vi "GEA3 Get ERD Info.vi"(4 "Enable EMV List":bool, 6 "Enable Heat Pump List":bool, 7 "Enable Inverter List":bool, 8 "error in (no error)":errorcluster, 9 "GEA Info?":bool, 11 "GEA3 Reference":refnum<k24>) -> (0 "error out":errorcluster, 2 "ERD Data":string[][](array[string]), 3 "ERD Data  2":T1)   [LabVIEW 2023]
uses:
  Type Definitions/GEA3 HEWH ERD Data.ctl
  Type Definitions/GEA3 HEWH Mixing Valve.ctl
  C:/TechnologyLab/NI-2010/Drivers/GEA3 Toolkit/GEA3 DLL Source/GeaCommunication.dll
  GEA3 DLL Source/GeaCommunication.dll
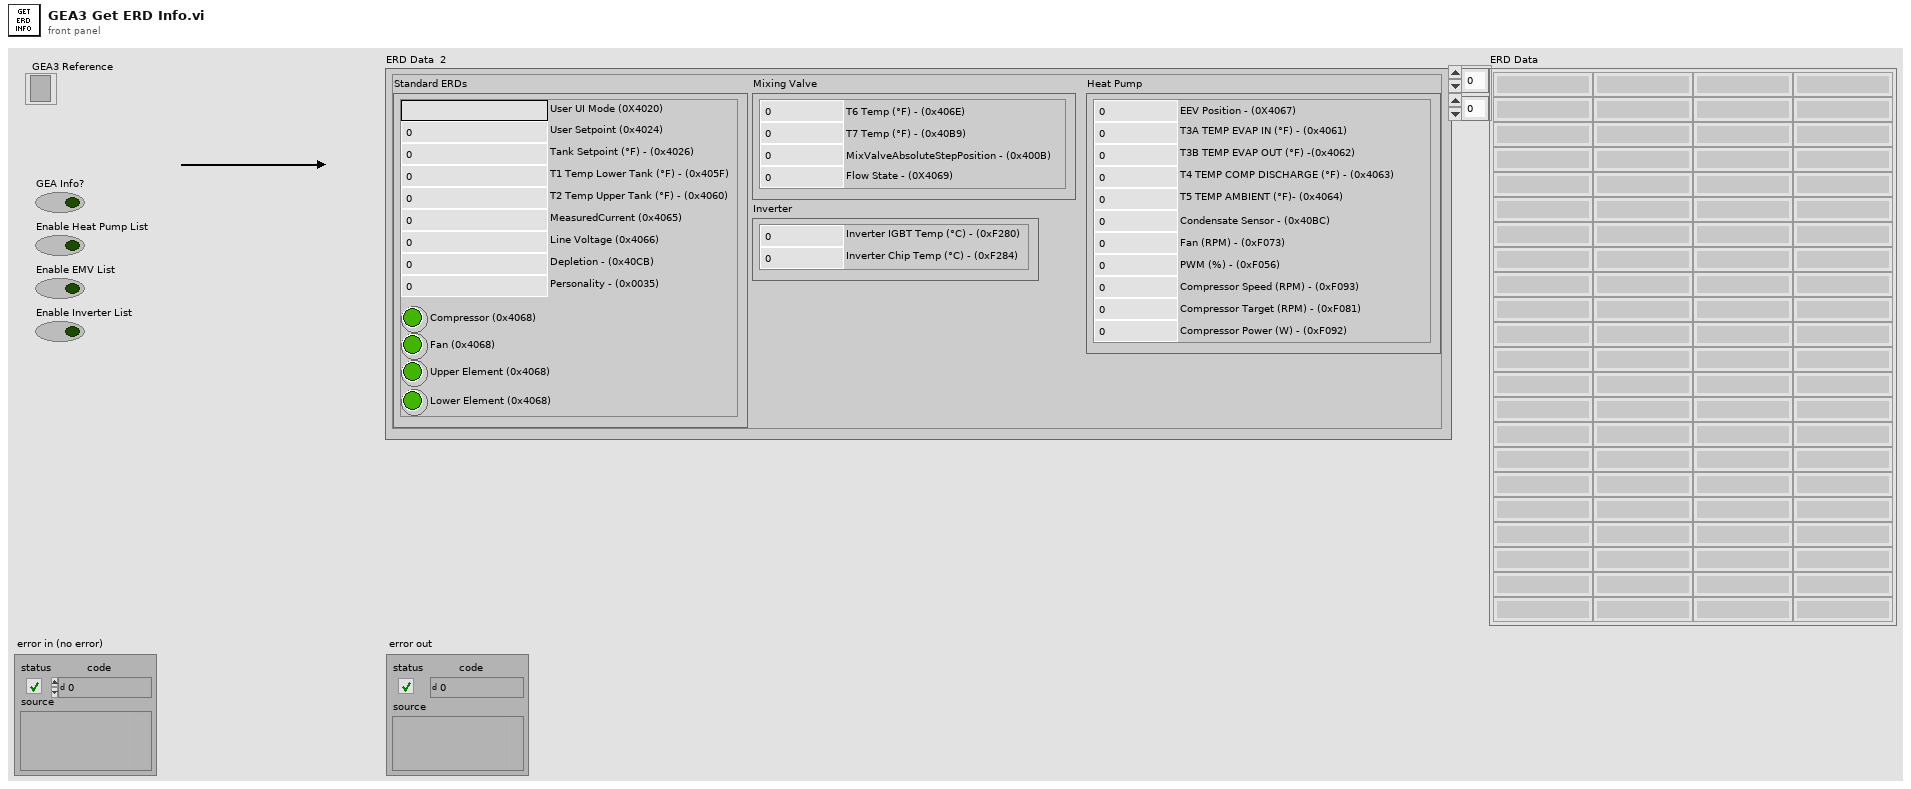
[diagram p1: front panel]
types:
  T1 = typedef "GEA3 HEWH ERD Data.ctl" = cluster{"Mixing Valve":T2, "Standard ERDs":cluster{"User UI Mode (0X4020)":string, "User Setpoint (0x4024)":u16, "Compressor (0x4068)":bool, "Lower Element (0x4068)":bool, "Upper Element (0x4068)":bool, "Fan (0x4068)":bool, "T1 Temp Lower Tank (°F) - (0x405F)":dbl, "T2 Temp Upper Tank (°F) - (0x4060)":dbl, "Line Voltage (0x4066)":u16, "MeasuredCurrent (0x4065)":dbl, "Tank Setpoint (°F) - (0x4026)":u16, "Depletion - (0x40CB)":u16, "Personality - (0x0035)":u16}, "Heat Pump":cluster{"EEV Position - (0X4067)":u16, "T3A TEMP EVAP IN (°F) - (0x4061)":dbl, "T3B TEMP EVAP OUT (°F) -(0x4062)":dbl, "T4 TEMP COMP DISCHARGE (°F) - (0x4063)":dbl, "T5 TEMP AMBIENT (°F)- (0x4064)":dbl, "Condensate Sensor - (0x40BC)":u16, "Fan (RPM) - (0xF073)":u16, "PWM (%) - (0xF056)":u16, "Compressor Speed (RPM) - (0xF093)":u16, "Compressor Target (RPM) - (0xF081)":u16, "Compressor Power (W) - (0xF092)":u16}, "Inverter":cluster{"Inverter IGBT Temp (°C) - (0xF280)":dbl, "Inverter Chip Temp (°C) - (0xF284)":dbl}}
  T2 = typedef "GEA3 HEWH Mixing Valve.ctl" = cluster{"T7 Temp (°F) - (0x40B9)":dbl, "MixValveAbsoluteStepPosition - (0x400B)":i16, "Flow State - (0X4069)":u8, "T6 Temp (°F) - (0x406E)":dbl}
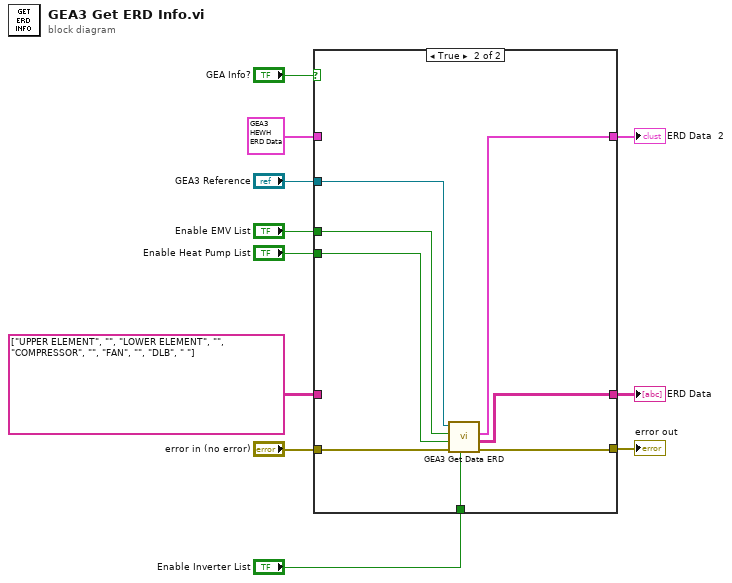
[diagram p0: block diagram]
diagram:
  n1 = case shown="True" "GEA Info?" {
    tunnel: "error in (no error)" -> [w14 w22]
    tunnel: [w14 w21] -> w2
    tunnel: "GEA3 Reference" -> [_ w20]
    tunnel: [w13 w19] -> w8
    tunnel: [w12 w18] -> w11
    tunnel: string[][] [["UPPER ELEMENT", ""], ["LOWER ELEMENT", ""], ["COMPRESSOR", ""], ["FAN", ""], ["DLB", " "]] ("ERD Data") -> [w13 _]
    tunnel: T1 {"Mixing Valve"={"T7 Temp (°F) - (0x40B9)"=0.0, "MixValveAbsoluteStepPosition - (0x400B)"=0, "Flow State - (0X4069)"=0, "T6 Temp (°F) - (0x406E)"=0.0}, "Standard ERDs"={"User UI Mode (0X4020)"="", "User Setpoint (0x4024)"=0, "Compressor (0x4068)"=FALSE, "Lower Element (0x4068)"=FALSE, "Upper Element (0x4068)"=FALSE, "Fan (0x4068)"=FALSE, "T1 Temp Lower Tank (°F) - (0x405F)"=0.0, "T2 Temp Upper Tank (°F) - (0x4060)"=0.0, "Line Voltage (0x4066)"=0, "MeasuredCurrent (0x4065)"=0.0, "Tank Setpoint (°F) - (0x4026)"=0, "Depletion - (0x40CB)"=0, "Personality - (0x0035)"=0}, "Heat Pump"={"EEV Position - (0X4067)"=0, "T3A TEMP EVAP IN (°F) - (0x4061)"=0.0, "T3B TEMP EVAP OUT (°F) -(0x4062)"=0.0, "T4 TEMP COMP DISCHARGE (°F) - (0x4063)"=0.0, "T5 TEMP AMBIENT (°F)- (0x4064)"=0.0, "Condensate Sensor - (0x40BC)"=0, "Fan (RPM) - (0xF073)"=0, "PWM (%) - (0xF056)"=0, "Compressor Speed (RPM) - (0xF093)"=0, "Compressor Target (RPM) - (0xF081)"=0, "Compressor Power (W) - (0xF092)"=0}, "Inverter"={"Inverter IGBT Temp (°C) - (0xF280)"=0.0, "Inverter Chip Temp (°C) - (0xF284)"=0.0}} ("ERD Data  2") -> [w12 _]
    tunnel: "Enable EMV List" -> [_ w17]
    tunnel: "Enable Heat Pump List" -> [_ w16]
    tunnel: "Enable Inverter List" -> [_ w15]
    frame False {
    }
    frame True {
      n2 = call "GEA3 Get Data ERD.vi"("Enable Inverter ERD List"=w15, "error in (no error)"=w22, "Enable Heat Pump List"=w16, "Enable EMV List"=w17, ".NET Refnum in"=w20) -> ("error out"=w21:errorcluster, "ERD Data"=w19:string[][], "ERD Data Input"=w18:T1)  [unwired: 3 in, 1 out]
    }
  }
  "ERD Data  2" <- w11
  "ERD Data" <- w8
  "error out" <- w2
